vi "disable driver after move.vi"(4 "channel number":string, 5 "Msg in":T1, 6 "channel index":i32, 7 "Numeric":i32, 8 "error in (no error)":errorcluster, 9 "Device and Axis":string, 10 "VISA resource name in":refnum<visa-resource-name>, 11 "ZaberASeries in":refnum<class "ZaberASeries.lvclass">) -> (0 "error out":errorcluster, 2 "VISA resource name out":refnum<visa-resource-name>, 3 "ZaberASeries out":refnum<class "ZaberASeries.lvclass">)   [LabVIEW 2020, in "ZaberASeries.lvclass"]
uses:
  ZaberASeries.lvclass
  BaseDriver/DriverMsg.ctl
  ZaberASeries.lvclass/ZaberASeries.ctl
  shared/OnOffTypeDef.ctl
  shared/CompressAndUpdate(Poly)/CompressAndUpdate(Enum).vi
  Zaber A Series.lvlib
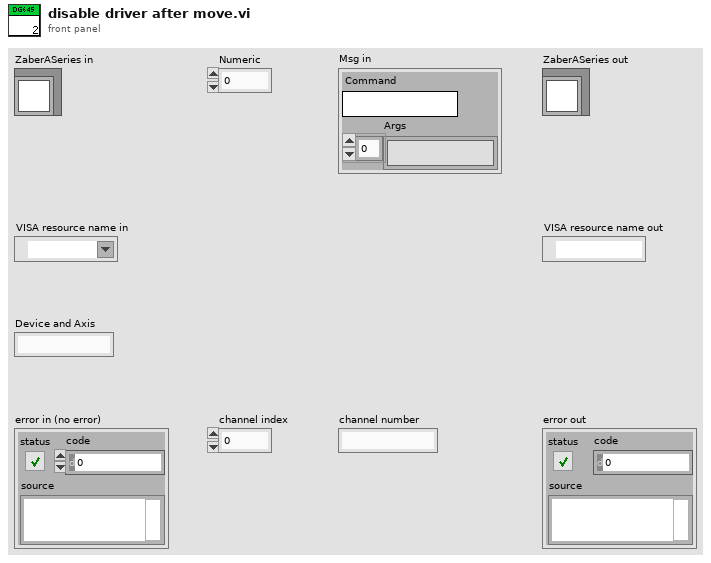
[diagram p1: front panel]
types:
  T1 = typedef "DriverMsg.ctl" = cluster{"Command":string, "Args":string[]}
  T2 = typedef "OnOffTypeDef.ctl" = enum16{"off", "on"}
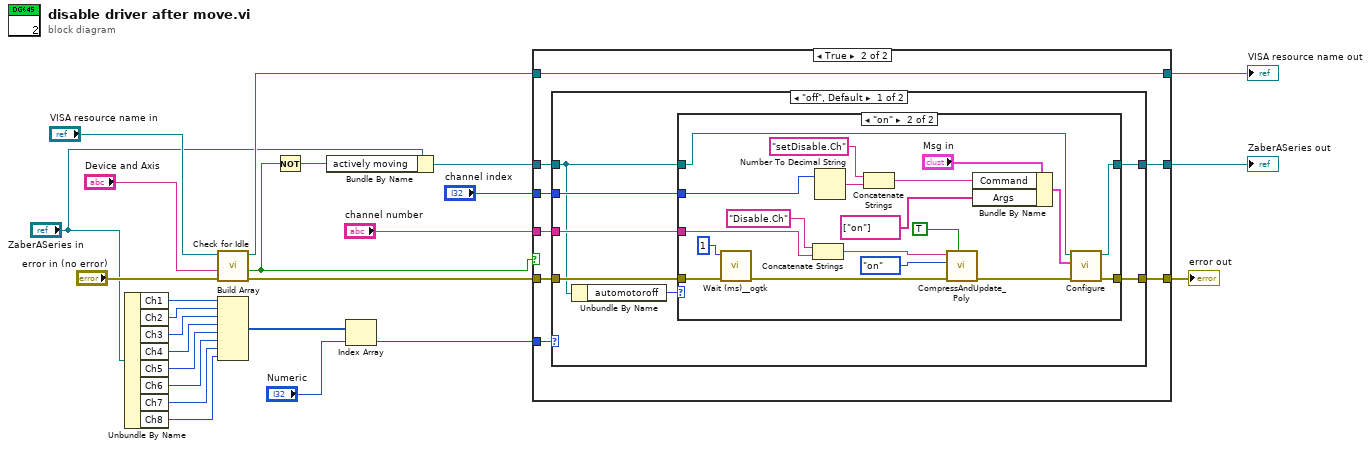
[diagram p0: block diagram]
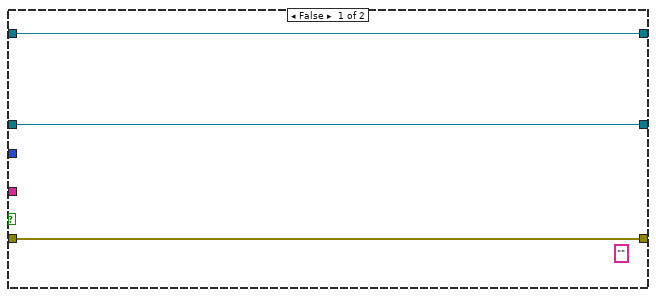
[diagram p2: hidden frame]
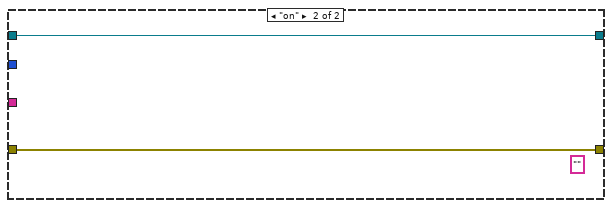
[diagram p4: hidden frame]
diagram:
  n1 = Unbundle By Name("ZaberASeries in") -> ("Ch1"=w21:T2, "Ch2"=w20:T2, "Ch3"=w19:T2, "Ch4"=w18:T2, "Ch5"=w4:T2, "Ch6"=w3:T2, "Ch7"=w2:T2, "Ch8"=w1:T2)
  n2 = call "Check for Idle.vi"("error in (no error)"="error in (no error)", "Device and Axis"="Device and Axis", "VISA resource name"="VISA resource name in") -> ("error out"=w22:errorcluster, "Idle"=w6:bool, "VISA resource name out"=w14:refnum<visa-resource-name>)  [unwired: 6 in]
  n3 = Build Array(w21, w20, w19, w18, w4, w3, w2, w1) -> (w17:T2[])
  n4 = Not(x=w6) -> (.not. x?=w5:bool)
  n5 = Bundle By Name(cluster="ZaberASeries in", "actively moving"=w5) -> (w7:refnum<class "ZaberASeries.lvclass">)
  n6 = Index Array(array=w17, index="Numeric") -> (element=w24:T2)
  n7 = case shown="True" w6 {
    tunnel: w22 -> [w28 w33]
    tunnel: [w28 w35] -> w12
    tunnel: [w27 w36] -> w13
    tunnel: w14 -> [w27 w36]
    tunnel: "channel index" -> [_ w34]
    tunnel: w24 -> [_ w32]
    tunnel: "channel number" -> [_ w31]
    tunnel: w7 -> [w26 w30]
    tunnel: [w26 w29] -> w25
    frame False {
      (unwired) "" ("new commands")
    }
    frame True {
      n8 = case shown="\"off\", Default" w32 {
        tunnel: [w40 w66] -> w35
        tunnel: w34 -> [w43 _]
        tunnel: w33 -> [w42 w66]
        tunnel: w31 -> [w41 _]
        tunnel: w30 -> [w38 w65]
        tunnel: [w39 w65] -> w29
        frame "off", Default {
          n9 = Unbundle By Name(w38) -> ("automotoroff"=w37:T2)
          n10 = case shown="\"on\"" w37 {
            tunnel: w43 -> [_ w62]
            tunnel: w42 -> [w45 w61]
            tunnel: w41 -> [_ w57]
            tunnel: [w45 w53] -> w40
            tunnel: w38 -> [w44 w52]
            tunnel: [w44 w51] -> w39
            frame "off", Default {
            }
            frame "on" {
              n11 = call <userlib>:"Wait (ms)__ogtk.vi"("error in (no error)"=w61, "milliseconds to wait"=u32 1) -> ("error out"=w55:errorcluster)  [unwired: 8 in, 1 out]
              n12 = Concatenate Strings("Disable.Ch" ("command or variable name"), w57) -> (w59:string)
              n13 = Number To Decimal String(number=w62) -> (decimal integer string=w63:string)  [unwired: 1 in]
              n14 = Concatenate Strings("setDisable.Ch" ("string"), w63) -> (w48:string)
              n15 = call-poly "CompressAndUpdate_Poly.vi"("force CVT update (false)"=TRUE, "error in"=w55, "enum variant"=OnOffTypeDef."on" ("Ch4"), "command or variable name"=w59) -> ("error out"=w54:errorcluster)  [unwired: 7 in]
              n16 = Bundle By Name(cluster="Msg in", "Command"=w48, "Args"=string[] ["on"]) -> (w47:T1)
              n17 = call-dynamic "Configure.vi"("error in (no error)"=w54, "Msg in"=w47, "ZaberASeries in"=w52) -> ("error out"=w53:errorcluster, "ZaberASeries out"=w51:refnum<class "ZaberASeries.lvclass">)  [unwired: 5 in, 2 out]
            }
          }
        }
        frame "on" {
          (unwired) "" ("new commands")
        }
      }
    }
  }
  "ZaberASeries out" <- w25
  "VISA resource name out" <- w13
  "error out" <- w12
